vi "IVCurvePulsed.vi"(5 "XYGraph Refnum":refnum<vi>, 6 "Status":refnum<vi>, 7 "Source Code":string="-- The local functions are scoped at the project level, so that we can keep\n-- track of the reading buffers throughout the test.\nreset()\nsmua.reset()\nlocal systemNodes = {}\nlocal systemSmus = {}\nlocal systemSmuReadingBufferIndexes = {}\nlocal appendMode = 1\nlocal rangei = 1e-3\nlocal doCap =0\nlocal gOverrunDetected = false\n-- ==========================================================================\n-- This function tests for overruns in any of the system smus' trigger models.\n-- It returns an error to the application that will be displayed in a\n-- dialog box if an overrun occurs.\n-- ==========================================================================\nlocal _Overruncheck = function()\n    -- ==========================================================================\n    -- This function test the results of the value in the smu's trigger overrun\n    -- status register. -- It returns an error if an overrun occurs.\n    --\n    -- parameter   overrun     A bit pattern that contains the smu trigger overrun\n    --                         status register result\n    -- ==========================================================================\n    local TestOverrunBits = function(overrun, selNode, whichSmu)\n        local whichNode = [[localnode.]]\n        if (selNode.tsplink.node ~= localnode.tsplink.node) then\n            whichNode = [[node[]] .. selNode.tsplink.node .. [[].]]\n        end\n        whichNode = whichNode .. whichSmu .. [[ (]] .. selNode.model .. [[)]]\n        if (bit.test(overrun, 2)) then\n            gOverrunDetected = true\n            return (\"arm overrun on \" .. whichNode .. \"{eol}\")\n        elseif (bit.test(overrun, 3)) then\n            gOverrunDetected = true\n            return (\"source overrun on \" .. whichNode .. \"{eol}\")\n        elseif (bit.test(overrun, 4)) then\n            gOverrunDetected = true\n            return (\"measure overrun on \" .. whichNode .. \"{eol}\")\n        elseif (bit.test(overrun, 5)) then\n            gOverrunDetected = true\n            return (\"end pulse overrun on \" .. whichNode .. \"{eol}\")\n        else\n            return (\"\")\n        end\n    end\n\n    -- Report an overrun error only once.\n    if (gOverrunDetected == false) then\n        local allSmusInOverrun = [[]]\n\n        for i, selNode in ipairs(systemNodes) do\n            for j, selSmu in ipairs(systemSmus[i]) do\n                if (j == 1) then\n                    local overrun = selNode.status.operation.instrument.smua.trigger_overrun.event\n                    if (overrun > 0) then\n                        allSmusInOverrun = allSmusInOverrun .. TestOverrunBits(overrun, selNode, [[smua]])\n                    end\n                elseif (j == 2) then\n                    local overrun = selNode.status.operation.instrument.smub.trigger_overrun.event\n                    if (overrun > 0) then\n                        allSmusInOverrun = allSmusInOverrun .. TestOverrunBits(overrun, selNode, [[smub]])\n                    end\n                end\n            end\n        end\n\n        if (gOverrunDetected == true) then\n            print(\"[{error}]Script stopped due to:{eol}\" .. allSmusInOverrun)\n        end\n    end\nend\n\nlocal gComplianceDetected = false\n-- ==========================================================================\n-- Checks smus for voltage or current compliance.\n-- If a compliance event occurs, the message dialog box is presented to the\n-- user.\n-- ==========================================================================\nlocal _ComplianceCheck = function()\n    -- Report a compliance error only once.\n    if (gComplianceDetected == false) then\n        local allSmusInCompliance = [[]]\n\n        for i, selNode in ipairs(systemNodes) do\n            for j, selSmu in ipairs(systemSmus[i]) do\n                local compDetect = selNode.status.measurement.instrument.event\n                if (compDetect > 0) then\n                    -- Compose and show error message\n                    local whichNode = [[localnode.]]\n                    if (selNode.tsplink.node ~= localnode.tsplink.node) then\n                        whichNode = [[node[]] .. selNode.tsplink.node .. [[].]]\n                    end\n                    local whichSmu = [[]]\n                    if (compDetect == 2) then\n                        whichSmu = whichNode .. [[smua]]\n                    elseif (compDetect == 4) then\n                        whichSmu = whichNode .. [[smub]]\n                    elseif (compDetect == 6) then\n                        whichSmu = whichNode .. [[smua and ]] .. whichNode .. [[smub]]\n                    end\n                    whichSmu = whichSmu .. [[ (]] .. selNode.model .. [[){eol}]]\n                    allSmusInCompliance = allSmusInCompliance .. whichSmu\n\n                    -- Set gComplianceDetected so we don't report the error again.\n                    gComplianceDetected = true\n                end\n            end\n        end\n\n        if (gComplianceDetected == true) then\n            print(\"[{info}]Compliance detected on:{eol}\" .. allSmusInCompliance ..\n                      \"{eol}Click the Advanced button and check the Source Limit setting.\")\n        end\n    end\nend\n\nlocal gTestAborted = false\n-- ==========================================================================\n-- This function waits up to a specified period for the sweeps to complete.\n-- If the delay parameter is -1, then the timeout is infinite. It returns true\n-- if all sweeping actions are complete. Otherwise, the return value is false.\n-- Note: If gTestAborted is true, this function returns false immediately.\n--\n-- parameter  interval     Maximum time to wait (in seconds).\n-- ==========================================================================\nlocal _WaitForComplete = function(interval)\n    local pollInterval = 0.1\n\n    -- ==========================================================================\n    -- Checks the system smus for any that are still sweeping.\n    -- ==========================================================================\n    local IsSweepingComplete = function()\n        for i, selNode in ipairs(systemNodes) do\n            for j, selSmu in ipairs(systemSmus[i]) do\n                if (j == 1) then\n                    local statcond = selNode.status.operation.instrument.smua.condition\n                    if (bit.test(statcond, 4)) then\n                        return false\n                    end\n                elseif (j == 2) then\n                    local statcond = selNode.status.operation.instrument.smub.condition\n                    if (bit.test(statcond, 4)) then\n                        return false\n                    end\n                end\n            end\n        end\n\n        return true\n    end\n\n    local notimeout = false\n    if (interval < 0) then\n        notimeout = true\n        interval = 1\n    end\n\n    while (interval > 0) do\n        -- Check the abort flag\n        if (gTestAborted == true) then\n            return false\n        end\n\n        -- Check for errors\n        if (errorqueue.count > 0) then\n            return false\n        end\n\n        -- Check for overruns and compliance\n        _Overruncheck()\n        _ComplianceCheck()\n\n        if (IsSweepingComplete() == true) then\n            return true\n        end\n\n        delay(pollInterval)\n\n        if (notimeout == false) then\n            interval = interval - pollInterval\n        end\n    end\n\n    if (IsSweepingComplete() == true) then\n        return true\n    end\n\n    return false\nend\n----------------------------------------------------------------------------\n-- START OF INITIALIZE SEGMENT ... do not modify this section\n----------------------------------------------------------------------------\n-- ==========================================================================\n-- This function prepares the test for execution. \n-- It first verifies that current setup matches project's setup. \n-- Then, it initializes members used to keep track of reading buffer storage.\n-- ==========================================================================\nfunction _Initialize()\n    local maxNodes = 64 -- Maximum possible nodes in TSP link system.\n\n    local projectSetup = {{localnode, [[2636A]], [[2.2.1]]}} -- Instrument configuration for the project.\n    local currentSetup = {} -- Current instrument configuration.\n\n    local errorTag = \"[{error}]\"\n    local errorMessage = {[[Instrument in project configuration not found.]],\n                          [[Instrument configuration at does not match.]]}\n    local errorNo = 0\n\n    -- ==========================================================================\n    -- Configures the status model to detect voltage or current compliance.\n    -- ==========================================================================\n    local ConfigStatusModel = function()\n        for i, selNode in ipairs(systemNodes) do\n            selNode.status.reset()\n            for j, selSmu in ipairs(systemSmus[i]) do\n                -- The selSmu.source.compliance call will force an update\n                -- the condition register of the measurement.instrument.smuX to\n                -- update\n                local dum = selSmu.source.compliance\n                if (j == 1) then\n                    -- Clear the measurement.instrument.smua event register by reading its value\n                    dum = selNode.status.measurement.instrument.smua.event\n                    -- Now configure the status model to detect voltage or current compliance\n                    selNode.status.measurement.instrument.smua.enable = 3\n                    selNode.status.measurement.instrument.smua.ptr = 3\n                    selNode.status.measurement.instrument.enable = 6\n                    selNode.status.measurement.instrument.ptr = 6\n                elseif (j == 2) then\n                    -- Clear the measurement.instrument.smub event register by reading its value\n                    dum = selNode.status.measurement.instrument.smub.event\n                    -- Now configure the status model to detect voltage or current compliance\n                    selNode.status.measurement.instrument.smub.enable = 3\n                    selNode.status.measurement.instrument.smub.ptr = 3\n                end\n            end\n        end\n    end\n\n    -- ==========================================================================\n    -- Determines the current system configuration.\n    -- ==========================================================================\n    local GetSetup = function()\n        local masterNode = tsplink.node\n\n        systemSmus = {}\n        systemNodes = {}\n        systemNodes[1] = node[masterNode]\n\n        currentSetup[1] = {}\n        currentSetup[1][1] = node[masterNode]\n        currentSetup[1][2] = node[masterNode].model\n        currentSetup[1][3] = node[masterNode].revision\n\n        systemSmus[1] = {}\n        systemSmus[1][1] = node[masterNode].smua\n\n        if (node[masterNode].smub ~= nil) then\n            systemSmus[1][2] = node[masterNode].smub\n        end\n\n        local j = 2\n        for i = 1, maxNodes do\n            if ((tsplink.node ~= i) and (node[i] ~= nil)) then\n                systemNodes[j] = node[i]\n                currentSetup[j] = {}\n                currentSetup[j][1] = node[i]\n                currentSetup[j][2] = node[i].model\n                currentSetup[j][3] = node[i].revision\n\n                systemSmus[j] = {}\n                systemSmus[j][1] = node[i].smua\n\n                if (node[i].smub ~= nil) then\n                    systemSmus[j][2] = node[i].smub\n                end\n                j = j + 1\n            end\n        end\n    end\n\n    GetSetup()\n\n    -- Check the project setup versus the configuration setup.\n    -- If there is a difference, report an error.\n    local numpInstruments = table.getn(projectSetup)\n    local numcInstruments = table.getn(currentSetup)\n\n    for i = 1, numpInstruments do\n        local pfields = table.getn(projectSetup[i])\n\n        errorNo = 1\n        for j = 1, numcInstruments do\n            -- Compare nodes.\n            if (projectSetup[i][1] == currentSetup[j][1]) then\n                errorNo = 0\n\n                for k = 2, pfields do\n                    if (projectSetup[i][k] ~= currentSetup[j][k]) then\n                        errorNo = 2\n                    end\n                end\n                break\n            end\n        end\n\n        if (errorNo > 0) then\n            break\n        end\n    end\n\n    if (errorNo > 0) then\n        error(errorMessage[errorNo])\n        print(errorTag .. errorMessage[errorNo])\n    end\n\n    -- ==========================================================================\n    -- Initializes all system readings buffers by clearing and setting them to\n    -- append mode. An array, sysSmuReadingBufferIndexes, is used to keep track of the\n    -- data stored to each of the reading buffers.\n    -- ==========================================================================\n    local InitalizeReadingBuffers = function()\n        systemSmuReadingBufferIndexes = {}\n        for i, selNode in ipairs(systemSmus) do\n            systemSmuReadingBufferIndexes[i] = {}\n\n            for j, selSmu in ipairs(selNode) do\n                -- Create an array for the smu.\n                systemSmuReadingBufferIndexes[i][j] = {}\n\n                local snvBuffers = {selSmu.nvbuffer1, selSmu.nvbuffer2}\n                for k, selBuffer in ipairs(snvBuffers) do\n                    -- Create an array for nvbuffers 1 and 2.\n                    systemSmuReadingBufferIndexes[i][j][k] = {}\n\n                    local sysSmuReadingBufferIndexes = systemSmuReadingBufferIndexes[i][j][k]\n                    sysSmuReadingBufferIndexes[\"start\"] = 0\n                    sysSmuReadingBufferIndexes[\"stop\"] = 0\n\n                    selBuffer.clear()\n                    selBuffer.appendmode = 1\n                    selBuffer.collecttimestamps = 1\n                    selBuffer.collectsourcevalues = 1\n                    selBuffer.timestampresolution = 1e-6\n                    if (selBuffer.fillmode ~= nil) then\n                        selBuffer.fillmode = selSmu.FILL_ONCE\n                    end\n                end\n\n            end\n        end\n    end\n\n    InitalizeReadingBuffers()\n    ConfigStatusModel()\nend\n----------------------------------------------------------------------------\n-- END OF INITIALIZE SEGMENT ... do not modify code after this point\n----------------------------------------------------------------------------\n\n----------------------------------------------------------------------------\n-- START OF SWEEP SEGMENT ... do not modify this section\n----------------------------------------------------------------------------\n-- ==========================================================================\n-- Configures a sweeping test.\n-- (This represents a Sweep segment of the script.  Click on the Sweep tab to customize it.)\n-- ==========================================================================\nfunction _Sweep()\n    local highSpeedSampling = false\n    local errorTag = \"[{error}]\"\n    local biasIndex = 1\n    local stepIndex = 2\n    local sweepIndex = 3\n    local numLevels = 3\n    local nvBuffersUsed = {1, 1, 1}\n    -- local alias for SMUs\n    local sweep1 = localnode.smua -- is a 2636A\n    -- \"NoStepFixed\" configuration (autorange enabled = false,  #step channels = 0):\n    -- This function configures any number of sweeping smus with no stepping smus.\n    -- It supports sweeps with autorange off and pulse mode.\n    local testSmus = {{{}}, -- Bias\n    {{}}, -- Step\n    {{localnode.smua}} -- Sweep\n    }\n\n    local testNodes = {{}, -- Bias\n    {}, -- Step\n    {localnode} -- Sweep\n    }\n\n    local sweepPulseModes = {{false}}\n\n    local timePoint = 0.1\n    local pulseWidth = 99.0000009537E-3\n    local measurePointTime = 16.7266666667E-3\n\n    local numberOfSteps = 1\n    local numberOfSweeps = #NumPoints\n\n    local nplc = 1\n    local lineFrequency = 60\n\n    local numNodes = table.getn(testNodes[sweepIndex])\n    local numMasterSmus = table.getn(testSmus[sweepIndex][1])\n    local masterNode = testNodes[sweepIndex][1]\n    local masterSweepSmu = testSmus[sweepIndex][1][1]\n\n    local t1Timer = masterNode.trigger.timer[1] -- t1Timer is for sweep time per point\n    local t2Timer = masterNode.trigger.timer[2] -- t2Timer is for sweep pulse width\n    local t3Timer = masterNode.trigger.timer[3] -- t3Timer is for a 1ms initial delay\n\n    local masterTspLine1 = masterNode.tsplink.trigger[1] -- for source stimulus\n    local masterTspLine2 = masterNode.tsplink.trigger[2] -- for endpulse stimulus\n\n    -- ==========================================================================\n    -- This function checks for errors or conflicts in the test settings (timing, ranges, etc.)\n    -- ==========================================================================\n    local CheckSettings = function()\n        local measureDelay = timePoint - measurePointTime\n\n        local errorMsg = nil\n\n        -- Valid timing paramaters\n        -- None of these errors should appear to the user.\n        if (masterSweepSmu == nil) then\n            errorMsg = [[Must have at least one sweeping smu.]]\n        elseif (timePoint <= 0) then\n            errorMsg = [[timePoint <= 0]]\n        elseif (pulseWidth <= 0) then\n            errorMsg = [[pulseWidth <= 0]]\n        elseif (pulseWidth > timePoint) then\n            errorMsg = [[pulseWidth > timePoint]]\n        elseif (measureDelay < 0) then\n            errorMsg = [[timePoint too small, <= measurePointTime]]\n        end\n\n        if (errorMsg ~= nil) then\n            print(errorTag .. errorMsg)\n            error(errorMsg)\n        end\n    end\n\n    -- ==========================================================================\n    -- This function configures the trigger line interaction between the smus.\n    -- ==========================================================================\n    local ConfigureTriggerLines = function()\n        -- ==========================================================================\n        -- This function configures the timers that are used in the test.\n        -- ==========================================================================\n        local ConfigureSweepTimers = function()\n            -- t3Timer provides a 1ms initial delay following the masterSweepSmu's armed event ID.\n            -- This is to ensure that masterSweepSmu is fully ready for the first source stimulus.\n            t3Timer.stimulus = masterSweepSmu.trigger.ARMED_EVENT_ID\n            t3Timer.passthrough = false\n            t3Timer.delay = 1.0e-3\n            t3Timer.count = 1\n\n            if (numberOfSweeps > 1) then\n                t1Timer.stimulus = t3Timer.EVENT_ID\n                t1Timer.passthrough = true\n                t1Timer.delay = timePoint\n                t1Timer.count = numberOfSweeps - 1\n\n                t2Timer.stimulus = t1Timer.EVENT_ID\n            else\n                -- Cannot use t1Timer when numberOfSweeps <= 1\n                t2Timer.stimulus = t3Timer.EVENT_ID\n            end\n\n            t2Timer.passthrough = false\n            t2Timer.delay = pulseWidth\n            t2Timer.count = 1\n        end\n\n        -- ==========================================================================\n        -- This function configures the sweeping smus.\n        -- ==========================================================================\n        local ConfigureSweep = function()\n\n            -- ==========================================================================\n            -- This function configures all sweeping smus on the master node.\n            -- ==========================================================================\n            local ConfigureMasterNodeSweepSmus = function()\n                for i = 1, numMasterSmus do\n                    local pulseMode = sweepPulseModes[1][i]\n                    local selSmu = testSmus[sweepIndex][1][i]\n                    local sourceStimulus = masterTspLine1.EVENT_ID\n\n                    if (i == 1) then\n                        -- masterSweepSmu will be triggered by StartSweep()\n                        -- Use a dummy event ID as a place holder for the arm stimulus\n                        selSmu.trigger.arm.stimulus = masterNode.trigger.EVENT_ID\n                    else\n                        selSmu.trigger.arm.stimulus = 0\n                    end\n\n                    selSmu.trigger.source.stimulus = sourceStimulus\n                    selSmu.trigger.source.action = selSmu.ENABLE\n\n                    if ((pulseMode == true) and (pulseWidth < timePoint)) then\n                        selSmu.trigger.endpulse.stimulus = masterTspLine2.EVENT_ID\n                        selSmu.trigger.endpulse.action = selSmu.SOURCE_IDLE\n                    else\n                        selSmu.trigger.endpulse.stimulus = selSmu.trigger.MEASURE_COMPLETE_EVENT_ID\n                        selSmu.trigger.endpulse.action = selSmu.SOURCE_HOLD\n                    end\n\n                    if (highSpeedSampling == true) then\n                        selSmu.trigger.measure.stimulus = sourceStimulus\n                        selSmu.trigger.measure.action = selSmu.ASYNC\n\n                        -- Cannot collect source values when in asynchronous mode\n                        selSmu.nvbuffer1.collectsourcevalues = 0\n                        selSmu.nvbuffer2.collectsourcevalues = 0\n                    else\n                        selSmu.trigger.measure.stimulus = 0\n                        selSmu.trigger.measure.action = selSmu.ENABLE\n                    end\n\n                    selSmu.trigger.arm.count = numberOfSteps\n                    selSmu.trigger.count = numberOfSweeps\n                end\n            end\n\n            -- ==========================================================================\n            -- This function configures a sweeping smu on a remote node\n            --\n            -- parameter pulseMode      true for Pulse mode,  false otherwise.\n            -- parameter selNode        Node to which the smu belongs.\n            -- parameter selSmu         Smu to configure.\n            -- ==========================================================================\n            local ConfigureRemoteSweepSmu = function(pulseMode, selNode, selSmu)\n                local tspl1 = selNode.tsplink.trigger[1]\n                local tspl2 = selNode.tsplink.trigger[2]\n                local sourceStimulus = tspl1.EVENT_ID\n\n                selSmu.trigger.arm.stimulus = 0\n                selSmu.trigger.source.stimulus = sourceStimulus\n                selSmu.trigger.source.action = selSmu.ENABLE\n\n                if ((pulseMode == true) and (pulseWidth < timePoint)) then\n                    selSmu.trigger.endpulse.stimulus = tspl2.EVENT_ID\n                    selSmu.trigger.endpulse.action = selSmu.SOURCE_IDLE\n                else\n                    selSmu.trigger.endpulse.stimulus = selSmu.trigger.MEASURE_COMPLETE_EVENT_ID\n                    selSmu.trigger.endpulse.action = selSmu.SOURCE_HOLD\n                end\n\n                if (highSpeedSampling == true) then\n                    selSmu.trigger.measure.stimulus = sourceStimulus\n                    selSmu.trigger.measure.action = selSmu.ASYNC\n\n                    -- Cannot collect source values when in asynchronous mode\n                    selSmu.nvbuffer1.collectsourcevalues = 0\n                    selSmu.nvbuffer2.collectsourcevalues = 0\n                else\n                    selSmu.trigger.measure.stimulus = 0\n                    selSmu.trigger.measure.action = selSmu.ENABLE\n                end\n\n                selSmu.trigger.arm.count = numberOfSteps\n                selSmu.trigger.count = numberOfSweeps\n            end\n\n            -- ===========================\n            -- START of ConfigureSweep()\n            -- ===========================\n            -- Prepare a tsplink trigger line for source stimulus on the master node\n            masterTspLine1.mode = tsplink.TRIG_FALLING\n            masterTspLine1.pulsewidth = 1e-6\n            if (numberOfSweeps > 1) then\n                masterTspLine1.stimulus = t1Timer.EVENT_ID\n            else\n                masterTspLine1.stimulus = t3Timer.EVENT_ID\n            end\n\n            -- Prepare a tsplink trigger line for endpulse stimulus on the master node\n            masterTspLine2.mode = tsplink.TRIG_FALLING\n            masterTspLine2.pulsewidth = 1e-6\n            masterTspLine2.stimulus = t2Timer.EVENT_ID\n\n            -- Configure all sweep smus on the master node.\n            -- The master node contains the smu that kicks off the sweeps.\n            ConfigureMasterNodeSweepSmus()\n\n            -- Configure the sweeping smus on remote nodes\n            if (numNodes > 1) then\n                for i = 2, numNodes do\n                    -- For each remote node, configure the tsplink trigger lines\n                    local selNode = testNodes[sweepIndex][i]\n\n                    local tspl1 = selNode.tsplink.trigger[1]\n                    tspl1.mode = tsplink.TRIG_FALLING\n                    tspl1.pulsewidth = 1e-6\n                    tspl1.stimulus = 0\n\n                    local tspl2 = selNode.tsplink.trigger[2]\n                    tspl2.mode = tsplink.TRIG_FALLING\n                    tspl2.pulsewidth = 1e-6\n                    tspl2.stimulus = 0\n\n                    local sweepSmus = testSmus[sweepIndex]\n                    local numSmus = table.getn(sweepSmus[i])\n\n                    for j = 1, numSmus do\n                        -- For each sweeping smu on each remote node, configure the remote sweeping smu\n                        local extSmu = sweepSmus[i][j]\n                        local pulseMode = sweepPulseModes[i][j]\n\n                        ConfigureRemoteSweepSmu(pulseMode, selNode, extSmu)\n                    end\n                end\n            end\n        end\n\n        -- Configure timers and sweep trigger lines.\n        ConfigureSweepTimers()\n        ConfigureSweep()\n    end\n\n    -- ==========================================================================\n    -- This function kicks off the sweep.\n    -- ==========================================================================\n    local StartSweep = function()\n        masterSweepSmu.trigger.arm.set()\n    end\n    -- ==========================================================================\n    -- Resets all components that may be used in the test.\n    -- ==========================================================================\n    local Reset = function()\n        for i, selTest in ipairs(testSmus) do\n            for j, selNode in ipairs(testNodes[i]) do\n                if (selNode ~= nil) then\n                    -- Reset blenders\n                    local k = 1\n                    while (selNode.tsplink.trigger[k] ~= nil) do\n                        selNode.tsplink.trigger[k].reset()\n                        k = k + 1\n                    end\n\n                    k = 1\n                    while (selNode.trigger.blender[k] ~= nil) do\n                        selNode.trigger.blender[k].reset()\n                        k = k + 1\n                    end\n\n                    -- Reset Timers\n                    k = 1\n                    while (selNode.trigger.timer[k] ~= nil) do\n                        selNode.trigger.timer[k].reset()\n                        k = k + 1\n                    end\n                end\n            end\n\n            -- Reset Smus\n            for j, selNode in ipairs(selTest) do\n                for k, selSmu in ipairs(selNode) do\n                    if (selSmu ~= nil) then\n                        -- Resets all smus in the test.\n                        selSmu.reset()\n                    end\n                end\n            end\n        end\n    end\n\n    -- ==========================================================================\n    -- Turns all smus in the test on.\n    -- ==========================================================================\n    local TurnSmusOn = function()\n        for i, selTest in ipairs(testSmus) do\n            for j, selNode in ipairs(selTest) do\n                for k, selSmu in ipairs(selNode) do\n                    if (selSmu ~= nil) then\n                        if (selSmu.source.output ~= 1) then\n                            selSmu.source.output = 1\n                        end\n                    end\n                end\n            end\n        end\n    end\n\n    -- ==========================================================================\n    -- This function initiates the steping and sweeping smus.\n    -- ==========================================================================\n    local InitiateSmus = function()\n        for i = 2, numLevels do\n            for j, selNode in ipairs(testSmus[i]) do\n                for k, selSmu in ipairs(selNode) do\n                    if (selSmu ~= nil) then\n                        selSmu.trigger.initiate()\n                    end\n                end\n            end\n        end\n    end\n\n    -- ==========================================================================\n    -- This function determines the number of points that will be in the buffer at the end of the test.\n    -- ==========================================================================\n    local StoreReadingBufferIndexes = function()\n        -- ==========================================================================\n        -- Determines reading buffer starting and stopping indexes.\n        -- parameter    testLevel    Index referring to bias, step, or sweep.\n        -- parameter    i            Node index.\n        -- parameter    selSmuIndex  Selected smu index.\n        -- ==========================================================================\n        local SetupLastPoints = function(testLevel, i, selSmuIndex)\n            local stoppingPoint1 = 0\n            local stoppingPoint2 = 0\n            local incVal = 0\n            local selSmuRbIndex1 = systemSmuReadingBufferIndexes[i][selSmuIndex][1]\n            local selSmuRbIndex2 = systemSmuReadingBufferIndexes[i][selSmuIndex][2]\n\n            selSmuRbIndex1[\"start\"] = 1\n            selSmuRbIndex2[\"start\"] = 1\n\n            -- appendMode is a local variable common to the script.\n            if (appendMode == 1) then\n                stoppingPoint1 = selSmuRbIndex1[\"stop\"]\n                stoppingPoint2 = selSmuRbIndex2[\"stop\"]\n            end\n            -- Bias setup\n            if (testLevel == biasIndex) then\n                incVal = 1\n                -- Step setup\n            elseif (testLevel == stepIndex) then\n                incVal = (1 * 1)\n                -- Sweep setup\n            elseif (testLevel == sweepIndex) then\n                if (highSpeedSampling == true) then\n                    incVal = (1 * 200 * 60)\n                else\n                    incVal = (1 * 200 * 1)\n                end\n            end\n\n            selSmuRbIndex1[\"stop\"] = stoppingPoint1 + incVal\n            if (nvBuffersUsed[testLevel] == 2) then\n                selSmuRbIndex2[\"stop\"] = stoppingPoint2 + incVal\n            end\n        end\n\n        for i, selTest in ipairs(testSmus) do\n            for j, selNode in ipairs(selTest) do\n                for k, selSmu in ipairs(selNode) do\n                    for l, selSysNode in ipairs(systemSmus) do\n                        if (selSysNode[1] == selSmu) then\n                            SetupLastPoints(i, l, 1)\n                        end\n\n                        if (selSysNode[2] ~= nil) then\n                            if (selSysNode[2] == selSmu) then\n                                SetupLastPoints(i, l, 2)\n                            end\n                        end\n                    end\n                end\n            end\n        end\n    end\n    ---==========================================================================\n    -- The following makes sure we capture a measurement from the bias channels\n    -- ==========================================================================\n    local MeasureBiasChannels = function()\n    end\n    -- ==========================================================================\n    -- This function Configures the smu options such as nplc, function, range, etc.\n    -- ==========================================================================\n    local ConfigureSmus = function(rangei)\n        -- set up Sweep (inner sweep) for sweep1\n        sweep1.sense = sweep1.SENSE_LOCAL\n        sweep1.source.delay = 0\n        sweep1.measure.nplc = nplc\n        sweep1.measure.autozero = sweep1.AUTOZERO_OFF\n        sweep1.measure.count = 1\n        sweep1.measure.filter.enable = sweep1.FILTER_OFF\n        sweep1.measure.filter.type = sweep1.FILTER_MOVING_AVG\n        sweep1.measure.filter.count = 1\n        sweep1.measure.delay = 0\n        sweep1.measure.delayfactor = 1\n        sweep1.measure.analogfilter = 0\n        sweep1.source.func = sweep1.OUTPUT_DCVOLTS\n        if sweep1.source.highc == sweep1.ENABLE then\n            sweep1.source.highc = sweep1.DISABLE\n        end\n        sweep1.source.limiti = 10E-3\n        sweep1.trigger.source.limiti = sweep1.LIMIT_AUTO\n        sweep1.source.autorangev = 0\n        sweep1.source.rangev = 2\n        sweep1.trigger.source.listv({#VoltList})\n        sweep1.measure.autorangei = 0\n        sweep1.measure.rangei = rangei -- 100E-12\n        sweep1.measure.autorangev = sweep1.source.autorangev\n        if (sweep1.measure.autorangev == 0) then\n            sweep1.measure.rangev = sweep1.source.rangev\n        end\n        sweep1.trigger.measure.iv(sweep1.nvbuffer1, sweep1.nvbuffer2)\n        nvBuffersUsed[sweepIndex] = 2\n    end\n    -- Test starts here.\n\n    -- Make sure previous test is done.\n\n    _WaitForComplete(-1)\n\n    CheckSettings()\n    Reset()\n\n    smua.source.limiti = 1e-3\n    smua.source.levelv = .001\n    smua.source.output = 1\n    delay(.1)\n    local reading = smua.measure.i() * 2000\n\n    if (reading < rangei) then\n        rangei = rangei / 100\n        smua.source.output = 1\n        smua.source.limiti = 1e-3\n        smua.measure.rangei = rangei\n        smua.source.levelv = .001\n        delay(.1)\n        reading = smua.measure.i() * 2000\n        if (reading < rangei) then\n            rangei = rangei / 100\n            smua.source.output = 1\n            smua.source.limiti = 1e-3\n            smua.measure.rangei = rangei\n            smua.source.levelv = .001\n            delay(.1)\n            reading = smua.measure.i() * 2000\n            if (reading < rangei) then\n                rangei = rangei / 1000\n                doCap =1\n                smua.source.levelv = 0\n            end\n        end\n    end\n\n    ConfigureSmus(rangei)\n    ConfigureTriggerLines()\n\n    StoreReadingBufferIndexes()\n    TurnSmusOn()\n    MeasureBiasChannels()\n    smua.source.levelv = 0\n\n    InitiateSmus()\n    delay(1)\n    StartSweep()\nend\n----------------------------------------------------------------------------\n-- END OF SWEEP SEGMENT ... do not modify code after this point\n----------------------------------------------------------------------------\n\n----------------------------------------------------------------------------\n-- START OF DATAREPORT SEGMENT ... do not modify this section\n----------------------------------------------------------------------------\n-- ==========================================================================\n-- This script returns a series of reading buffers. \n-- (This represents a DataReport segment of the script.  Click on the Data tab to customize it.)\n-- ==========================================================================\nfunction _Data()\n    local buffers = {localnode.smua.nvbuffer1, localnode.smua.nvbuffer2} -- Array of reading buffers to return\n    local bufferNames = {[[localnode.smua.nvbuffer1]], [[localnode.smua.nvbuffer2]]} -- Array of reading buffer names\n    local bufferSmuNames = {[[Sweep_SMU]], [[Sweep_SMU]]} -- Array of SMU names for each reading buffer\n    local expectedCount = {} -- Array containing the expected number of return values.\n    local waitInterval = 1 -- Interval between message transfers\n    local maxToReturn = 100 -- Maximum reading buffer points between message transfers.\n\n    -- The following are special tokens used internally by the data report function\n    local DATA_REPORT = \"(({{Data}}))\"\n    local SWEEPSTART = \"{SWEEP-START}\"\n    local START = \"{START}\"\n    local NAME = \"{NAME}\"\n    local EXPECTED_COUNT = \"{EXPECTED-COUNT}\"\n    local PTS_IN_BUFF = \"{PTS-IN-BUFF}\"\n    local PTS_RETURNED = \"{PTS-RETURNED}\"\n    local BASE_TIME_STAMP = \"{BASE-TIME-STAMP}\"\n    local READINGS = \"{READINGS}\"\n    local TIMESTAMPS = \"{TIMESTAMPS}\"\n    local SRCVALS = \"{SRCVALS}\"\n    local END = \"{END}\"\n    local COMPLETE = \"{COMPLETE}\"\n\n    local errorTag = \"[{error}]\"\n    local dataIndexes = {} -- Data transfer index for each reading buffer\n    local done = true -- True when data transfer from all of reading buffers is completed\n    local dataComplete = true -- True when all of reading buffers have reached their expected counts\n\n    -- ==========================================================================\n    -- This function determines the ending points that will be in the buffer\n    -- at the time data collection takes place.\n    -- ==========================================================================\n    local GetStopPoints = function()\n        for i, selBuffer in ipairs(buffers) do\n            for j, selSysNode in ipairs(systemSmus) do\n                for k, selSmu in ipairs(selSysNode) do\n                    if (selSmu.nvbuffer1 == selBuffer) then\n                        expectedCount[i] = systemSmuReadingBufferIndexes[j][k][1][\"stop\"]\n                    elseif (selSmu.nvbuffer2 == selBuffer) then\n                        expectedCount[i] = systemSmuReadingBufferIndexes[j][k][2][\"stop\"]\n                    end\n                end\n            end\n        end\n    end\n\n    -- ==========================================================================\n    -- Checks if the SMU for selBuffer is sweeping.\n    -- ==========================================================================\n    local IsSweeping = function(selBuffer)\n        for i, selNode in ipairs(systemNodes) do\n            for j, selSmu in ipairs(systemSmus[i]) do\n                if (j == 1) then\n                    if ((selSmu.nvbuffer1 == selBuffer) or (selSmu.nvbuffer2 == selBuffer)) then\n                        local statcond = selNode.status.operation.instrument.smua.condition\n                        return (bit.test(statcond, 4)) -- Check Bit B3, Sweeping (SWE)\n                    end\n                elseif (j == 2) then\n                    if ((selSmu.nvbuffer1 == selBuffer) or (selSmu.nvbuffer2 == selBuffer)) then\n                        local statcond = selNode.status.operation.instrument.smub.condition\n                        return (bit.test(statcond, 4)) -- Check Bit B3, Sweeping (SWE)\n                    end\n                end\n            end\n        end\n        return false\n    end\n\n    -- ==========================================================================\n    -- Clears the reading buffers and resets the array that contains the\n    -- reading buffer storage start/ stop points.\n    -- ==========================================================================\n    local ClearReturnedBuffers = function()\n        for i, selBuffer in ipairs(buffers) do\n            selBuffer.clear()\n\n            local smuBufferIndex = nil\n            for j, selSysNode in ipairs(systemSmus) do\n                for k, selSmu in ipairs(selSysNode) do\n                    if (selSmu.nvbuffer1 == selBuffer) then\n                        smuBufferIndex = systemSmuReadingBufferIndexes[j][k][1]\n                    elseif (selSmu.nvbuffer2 == selBuffer) then\n                        smuBufferIndex = systemSmuReadingBufferIndexes[j][k][2]\n                    end\n                end\n            end\n            if (smuBufferIndex ~= nil) then\n                smuBufferIndex[\"start\"] = 0\n                smuBufferIndex[\"stop\"] = 0\n            end\n        end\n    end\n\n    GetStopPoints()\n\n    -- Initialize dataIndex. This array is used to keep track of the points returned to\n    -- the application.\n\n    for i, v in ipairs(buffers) do\n        dataIndexes[i] = 1\n    end\n\n    -- The following print statements turns on data report feature within the application.\n\n    repeat\n        done = true\n        dataComplete = true\n        for i, selBuffer in ipairs(buffers) do\n            -- Check for smu trigger model overruns.\n            _Overruncheck()\n\n            -- Check for smu compliance.\n            _ComplianceCheck()\n\n            -- Caution: Check for stillSweeping BEFORE getting numPointsStored\n            local stillSweeping = IsSweeping(selBuffer)\n            local numPointsStored = selBuffer.n\n\n            -- Check for sweep completion before data is complete (i.e. something bad happened)\n            if ((numPointsStored < expectedCount[i]) and (stillSweeping == false)) then\n                gTestAborted = true\n            end\n\n            dataComplete = dataComplete and (numPointsStored >= expectedCount[i])\n            done = done and (dataIndexes[i] > expectedCount[i])\n\n            if (dataIndexes[i] <= numPointsStored) then\n                local points = numPointsStored - dataIndexes[i] + 1\n\n                if (points > maxToReturn) then\n                    points = maxToReturn\n                end\n\n                local retString = string.format(\"%d,%d,\", i, points)\n\n                local start = dataIndexes[i]\n                local stop = start + points - 1\n\n                local readings = \"\"\n\n                for j = start, stop do\n                    if (j == start) then\n                        readings = readings .. string.format(\"%e,\", selBuffer.readings[j])\n                    else\n                        readings = readings .. string.format(\"%e,\", selBuffer.readings[j])\n                    end\n                end\n\n                local timestamps = \"\"\n                if (selBuffer.collecttimestamps == 1) then\n                    for j = start, stop do\n                        if (j == start) then\n                            timestamps = timestamps .. string.format(\"%e,\", selBuffer.timestamps[j])\n                        else\n                            timestamps = timestamps .. string.format(\"%e,\", selBuffer.timestamps[j])\n                        end\n                    end\n                end\n\n                local srcValues = \"\"\n                if (selBuffer.collectsourcevalues == 1) then\n                    for j = start, stop do\n                        if (j == start) then\n                            srcValues = srcValues .. string.format(\"%e,\", selBuffer.sourcevalues[j])\n                        else\n                            srcValues = srcValues .. string.format(\"%e,\", selBuffer.sourcevalues[j])\n                        end\n                    end\n                end\n\n                dataIndexes[i] = stop + 1\n\n                print(string.format(\"%d,%d,\", i + 1, points) .. readings)\n                print(string.format(\"%d,%d,\", 0, points) .. timestamps)\n                print(string.format(\"%d,%d,\", 1, points) .. srcValues)\n\n            end\n        end\n\n        if (dataComplete == false) then\n            if (gTestAborted == true) then\n                done = true -- Stop waiting for data completion because it will never happen\n            else\n                delay(waitInterval)\n            end\n        end\n    until (done == true)\n\n    print(COMPLETE .. \"\\n\")\n\n    -- The application may not have selected all the buffers being used in the test, so\n    -- we need to make sure the overlapped operations are complete before clearing the buffers.\n    local sweepCompleted = _WaitForComplete(-1)\n\n    if (sweepCompleted == true) then\n        ClearReturnedBuffers()\n    end\nend\n----------------------------------------------------------------------------\n-- END OF DATAREPORT SEGMENT ... do not modify code after this point\n----------------------------------------------------------------------------\n\n----------------------------------------------------------------------------\n-- START OF FINALIZE SEGMENT ... do not modify this section\n----------------------------------------------------------------------------\n-- ==========================================================================\n-- The function completes the script and places the instrument in a known state.\n-- ==========================================================================\nfunction _Finalize()\n    -- Wait for test completion\n    local sweepCompleted = _WaitForComplete(-1)\n\n    -- Check for abnornal completion\n    if (sweepCompleted == false) then\n        -- Abort all overlapped operations on all smus\n        for i, selNode in ipairs(systemNodes) do\n            for j, selSmu in ipairs(systemSmus[i]) do\n                selSmu.abort()\n            end\n        end\n\n        -- Check for errors\n        if (errorqueue.count > 0) then\n            print(\"[{error}]Script stopped due to error(s).\")\n        else\n            print(\"[{error}]Script stopped before completion.\")\n        end\n    end\n\n    -- Set output level to 0V and 0A for all SMUs\n    for i, selNode in ipairs(systemNodes) do\n        for j, selSmu in ipairs(systemSmus[i]) do\n            selSmu.source.leveli = 0\n            selSmu.source.levelv = 0\n        end\n    end\n\n    -- Turn output off for all SMUs\n    for i, selNode in ipairs(systemNodes) do\n        for j, selSmu in ipairs(systemSmus[i]) do\n            selSmu.source.output = 0\n        end\n    end\n\n    -- Reset the system,  placing it into a known safe state.\n    reset()\nend\n----------------------------------------------------------------------------\n-- END OF FINALIZE SEGMENT ... do not modify code after this point\n----------------------------------------------------------------------------\n\n_Initialize()\n_Sweep()\n_Data()\n_Finalize()\n\n\n\n\nfunction AC_Waveform_Sweep(Vrms,VLin, numCycles, frequency, limitI,skips)\n\treset()\n\tlocal COMPLETE = \"{COMPLETE}\"\n\t-- Generate the source values\n\tlocal Vpp\t\t\t\t= Vrms * math.sqrt(2)\n\tlocal sourceValues\t\t= {} \n\tlocal pointsPerCycle\t= 7200 / frequency\n\tlocal numDataPoints\t\t= pointsPerCycle * numCycles\n\n\tlocal res = {}\n    local cap = {}\n    for i = 1, numDataPoints do\n        res[i] = math.sin(i * 2 * math.pi / pointsPerCycle)\n        cap[i] = math.cos(i * 2 * math.pi / pointsPerCycle)\n        sourceValues[i] = (Vpp * res[i]) + Vpp + VLin\n    end\n\n\t-- Configure the SMU ranges\n\tsmua.reset()\n\tsmua.source.settling\t\t= smua.SETTLE_FAST_POLARITY\n\tsmua.source.autorangev\t\t= smua.AUTORANGE_OFF\n\tsmua.source.autorangei\t\t= smua.AUTORANGE_OFF\n\tsmua.source.rangev\t\t\t= 2 * Vpp + VLin\n\tsmua.source.delay\t\t\t= 0\n\tsmua.source.limiti\t\t\t= 1e-3\n\n\tsmua.measure.autorangev\t\t= smua.AUTORANGE_OFF\n\tsmua.measure.autorangei\t\t= smua.AUTORANGE_OFF\n\tsmua.measure.autozero\t\t= smua.AUTOZERO_OFF\n\tsmua.measure.delay\t\t\t= 0\n\tsmua.measure.delayfactor    = 1\n\tsmua.measure.analogfilter   = 0\n\n\t-- Voltage will be measured on the same range as the source range\n\tsmua.measure.rangei\t\t\t= limitI\n\tsmua.measure.nplc\t\t\t= 0.001\n\n\t-- Prepare the Reading Buffers\n\tsmua.nvbuffer1.clear()\n\tsmua.nvbuffer1.collecttimestamps\t= 1\n\tsmua.nvbuffer2.clear()\n\tsmua.nvbuffer2.collecttimestamps\t= 1\n\n\t-- Configure the trigger model\n\t--============================\n\t\n\t-- Timer 1 controls the time between source points\n\ttrigger.timer[1].delay = (1 / 7200)\n\ttrigger.timer[1].passthrough = true\n\ttrigger.timer[1].stimulus = smua.trigger.ARMED_EVENT_ID\n\ttrigger.timer[1].count = numDataPoints - 1\n\n\t-- Configure the SMU trigger model\n\tsmua.trigger.source.listv(sourceValues)\n\tsmua.trigger.source.limiti\t\t= limitI\n\tsmua.trigger.measure.action\t\t= smua.ENABLE\n\tsmua.trigger.measure.iv(smua.nvbuffer1, smua.nvbuffer2)\n\tsmua.trigger.endpulse.action\t= smua.SOURCE_HOLD\n\tsmua.trigger.endsweep.action\t= smua.SOURCE_IDLE\n\tsmua.trigger.count\t\t\t\t= numDataPoints\n\tsmua.trigger.arm.stimulus\t\t= 0\n\tsmua.trigger.source.stimulus\t= trigger.timer[1].EVENT_ID\n\tsmua.trigger.measure.stimulus\t= 0\n\tsmua.trigger.endpulse.stimulus\t= 0\n\tsmua.trigger.source.action\t\t= smua.ENABLE\n\t-- Ready to begin the test\n\n\tsmua.source.output\t\t\t\t\t= smua.OUTPUT_ON\n\t-- Start the trigger model execution\n\tsmua.trigger.initiate()\n\t-- Wait until the sweep has completed\n\twaitcomplete()\n\tsmua.source.output\t\t\t\t\t= smua.OUTPUT_OFF\n\n\t-- Print the data back to the Console in tabular format\n    singleWave = {}\n\tvisits ={}\n\tsize1=0\n\tphaseC = 0\n    phaseS = 0\n    mid = 0\n    cc=0\n    for x=pointsPerCycle, smua.nvbuffer2.n do\n      \tlocal i = math.floor( x - math.floor(x/(pointsPerCycle))*(pointsPerCycle))\n\t\tv=\tsmua.nvbuffer1[x]\n\t\tif (math.abs(v)<1e-3) then\n            if (singleWave[i]==nil) then \n                singleWave[i]=v\n                visits[i]=1\n                if (size1<i) then size1=i end\n            else \n                singleWave[i]=singleWave[i]+v\n                visits[i]=visits[i]+ 1\n            end\t\n        end\n\t\tphaseC = phaseC + cap[x] * v\n        phaseS = phaseS + res[x] * v\n        mid = mid + v\n        cc=cc+1\n--\t    print(smua.nvbuffer1.timestamps[x], smua.nvbuffer2[x], smua.nvbuffer1[x])\n    end\n\n    mid = mid / cc\n    phaseC = 2 * phaseC / cc\n    phaseS = 2 * phaseS / cc\n\n    rms=0\n    for x=pointsPerCycle, smua.nvbuffer2.n do\n      v=\tsmua.nvbuffer1[x]\n      rms=rms + (v-mid)*(v-mid)\n    end\n    rms = math.sqrt(rms/cc)\n\n    phase = 0\n    cc=0\n    for c=1,numCycles-1 do\n\t\tx0=pointsPerCycle*c\n\t\tfor x=x0+1,x0+pointsPerCycle-2 do\n             if ( smua.nvbuffer1[x]<=mid and  smua.nvbuffer1[x+1]>mid) then\n\t\t\t\tphase =phase + (x-x0)/pointsPerCycle\n                cc=cc+1\n\t\t\t\tbreak\n\t\t\t end\n\t\tend\n\tend\n   \n   pointsPerCycle=math.floor(pointsPerCycle)\n   omega=frequency*2*math.pi\n   print(frequency, VLin, Vpp, phaseC/Vpp* math.sqrt(omega) *1565856180.88521 -57.2098793899397 , rms/Vrms, phaseC/Vpp, phaseS/Vpp,rms,2*math.pi* phase/cc)\n  \nend\n\n\n\n\nfunction Square_Waveform_Sweep(Vrms, numCycles, frequency, limitI)\n    reset()\n    local COMPLETE = \"{COMPLETE}\"\n    -- Generate the source values\n    local Vpp = Vrms * math.sqrt(2)\n    local sourceValues = {}\n    local pointsPerCycle = 7200 / frequency\n    local numDataPoints = pointsPerCycle * numCycles\n\n    for i = 1, numDataPoints do\n        if ((Vpp * math.sin(i * 2 * math.pi / pointsPerCycle)) < 0) then\n            sourceValues[i] = Vpp\n        else\n            sourceValues[i] = 0\n        end\n    end\n\n    -- Configure the SMU ranges\n    smua.reset()\n    smua.source.settling = smua.SETTLE_FAST_POLARITY\n    smua.source.autorangev = smua.AUTORANGE_OFF\n    smua.source.autorangei = smua.AUTORANGE_OFF\n    smua.source.rangev = Vpp\n    smua.source.delay = 0\n    smua.source.limiti = 1e-12\n\n    smua.measure.autorangev = smua.AUTORANGE_OFF\n    smua.measure.autorangei = smua.AUTORANGE_OFF\n    smua.measure.autozero = smua.AUTOZERO_OFF\n    smua.measure.delay = 0\n    smua.measure.delayfactor = 1\n    smua.measure.analogfilter = 0\n\n    -- Voltage will be measured on the same range as the source range\n    smua.measure.rangei = limitI\n    smua.measure.nplc = 0.001\n\n    -- Prepare the Reading Buffers\n    smua.nvbuffer1.clear()\n    smua.nvbuffer1.collecttimestamps = 1\n    smua.nvbuffer2.clear()\n    smua.nvbuffer2.collecttimestamps = 1\n\n    -- Configure the trigger model\n    -- ============================\n\n    -- Timer 1 controls the time between source points\n    trigger.timer[1].delay = (1 / 7200)\n    trigger.timer[1].passthrough = true\n    trigger.timer[1].stimulus = smua.trigger.ARMED_EVENT_ID\n    trigger.timer[1].count = numDataPoints - 1\n\n    -- Configure the SMU trigger model\n    smua.trigger.source.listv(sourceValues)\n    smua.trigger.source.limiti = limitI\n    smua.trigger.measure.action = smua.ENABLE\n    smua.trigger.measure.iv(smua.nvbuffer1, smua.nvbuffer2)\n    smua.trigger.endpulse.action = smua.SOURCE_HOLD\n    smua.trigger.endsweep.action = smua.SOURCE_IDLE\n    smua.trigger.count = numDataPoints\n    smua.trigger.arm.stimulus = 0\n    smua.trigger.source.stimulus = trigger.timer[1].EVENT_ID\n    smua.trigger.measure.stimulus = 0\n    smua.trigger.endpulse.stimulus = 0\n    smua.trigger.source.action = smua.ENABLE\n    -- Ready to begin the test\n\n    smua.source.output = smua.OUTPUT_ON\n    -- Start the trigger model execution\n    smua.trigger.initiate()\n    -- Wait until the sweep has completed\n    waitcomplete()\n    smua.source.output = smua.OUTPUT_OFF\n\n    -- Print the data back to the Console in tabular format\n    singleWave = {}\n    visits = {}\n    size1 = 0\n    for x = 1, smua.nvbuffer2.n do\n        local i = math.floor(x - math.floor(x / (pointsPerCycle)) * (pointsPerCycle))\n        v = smua.nvbuffer1[x]\n        if (math.abs(v) < 1e-3) then\n            if (singleWave[i] == nil) then\n                singleWave[i] = v\n                visits[i] = 1\n                if (size1 < i) then\n                    size1 = i\n                end\n            else\n                singleWave[i] = singleWave[i] + v\n                visits[i] = visits[i] + 1\n            end\n        end\n        --    print(smua.nvbuffer1.timestamps[x], smua.nvbuffer2[x], smua.nvbuffer1[x],i,singleWave[i])\n    end\n\n    \n    maxV = 0\n    maxI = 0\n    timeI = 0\n    for x = 1, size1 do\n        singleWave[x] = singleWave[x] / visits[x]\n        v = smua.nvbuffer2[x + pointsPerCycle]\n        if (v > maxV) then\n            maxV = v\n        end\n        if (singleWave[x] > maxI) then\n            maxI = singleWave[x]\n            timeI = x\n        end\n    end\n\n    pointsPerCycle = math.floor(pointsPerCycle)\n    timeEnd =0\n    for x = timeI, size1 - 1 do\n        --print(smua.nvbuffer1.timestamps[x] - smua.nvbuffer1.timestamps[timeI], smua.nvbuffer2[x + pointsPerCycle],            singleWave[x] / maxI)\n        i = singleWave[x] / maxI\n        if (i < .36) then\n            timeEnd = smua.nvbuffer1.timestamps[x] - smua.nvbuffer1.timestamps[timeI]\n            break\n        end\n    end\n    \n    print(frequency, 0, Vpp, timeEnd/4031000 , maxI/Vpp, timeEnd,0,maxI,timeEnd)\n\nend\n\nif (doCap==1) then \n    AC_Waveform_Sweep(.01,0, 15, 30,  10e-9,10)\n    AC_Waveform_Sweep(.01,0, 30, 60,  10e-9,5)\n    AC_Waveform_Sweep(.01,0, 100, 200,  10e-9,1)\n    AC_Waveform_Sweep(.01,0, 150, 300,  10e-9,1)\n\n    AC_Waveform_Sweep(.01,-.1, 200, 400,  10e-9,1)\n    AC_Waveform_Sweep(.01,-.05, 200, 400,  10e-9,1)\n    AC_Waveform_Sweep(.01,0.0, 200, 400,  10e-9,1)\n    AC_Waveform_Sweep(.01,0.05, 200, 400,  10e-9,1)\n    AC_Waveform_Sweep(.01,0.1, 200, 400,  10e-9,1)\n\n    Square_Waveform_Sweep(.01, 40, 80,  10e-9)\nelse \n    for c=1,10 do\n        print(0, 0, 0, 0 , 0, 0,0,0,0)\n    end\nend\n\nprint(\"{COMPLETE}\")\n\n\n", 8 "CurrentRange":dbl=1e-10, 9 "Source Measure Unit Channel (0: Channel A)":i32, 10 "Waveform":waveform(dbl), 11 "VISA Refnum in":refnum<visa-resource-name>) -> (1 "appended array":dbl[][](array[numeric]), 3 "InfoCluster":T1)   [LabVIEW 2020]
uses:
  CapacitanceRecord.ctl
  CapacitanceInfos.ctl
  Keithley 2600 Series/Keithley 2600 Series.lvlib
panel:
  out "CapacitanceRecords":T2[](array[typedef])
  out "Device":dbl[][](array[numeric])=[[0.0, 0.099997, 0.199996, 0.299996, 0.399996, 0.499997, 0.599996, 0.699997, 0.799997, 0.899996, 0.0, 0.099997, 0.199996, 0.299996, 0.399996, 0.499997, 0.599996, 0.699997, 0.799997, 0.899996, 0.999996, 1.099997, 1.199997, 1.299996, 1.399996, 1.499996, 1.599996, 1.699996, 1.799996, 1.899996, 0.999996, 1.099997, 1.199997, 1.299996, 1.399996, 1.499996, 1.599996, 1.699996, 1.799996, 1.899996, 1.999996, 2.099996, 2.199997, 2.299996, 2.399996, 2.499997, 2.599997, 2.699996, 2.799996, 2.899997, 2.999996, 1.999996, 2.099996, 2.199997, 2.299996, 2.399996, 2.499997, 2.599997, 2.699996, 2.799996, 2.899997, 2.999996, 3.099996, 3.199996, 3.299997, 3.399996, 3.499997, 3.599996, 3.699996, 3.799997, 3.899996, 3.999997, 3.099996, 3.199996, 3.299997, 3.399996, 3.499997, 3.599996, 3.699996, 3.799997, 3.899996, 3.999997, 4.099997, 4.199996, 4.299997, 4.399996, 4.499997, 4.599997, 4.699996, 4.799996, 4.899996, 5.000106, 4.099997, 4.199996, 4.299997, 4.399996, 4.499997, 4.599997, 4.699996, 4.799996, 4.899996, 5.000106, 5.099996, 5.199996, 5.299997, 5.399996, 5.499996, 5.599996, 5.699996, 5.799997, 5.899997, 5.999996, 5.099996, 5.199996, 5.299997, 5.399996, 5.499996, 5.599996, 5.699996, 5.799997, 5.899997, 5.999996, 6.099997, 6.199997, 6.300001, 6.399997, 6.499996, 6.599996, 6.699996, 6.799996, 6.899996, 6.999996, 6.099997, 6.199997, 6.300001, 6.399997, 6.499996, 6.599996, 6.699996, 6.799996, 6.899996, 6.999996, 7.099996, 7.199997, 7.299996, 7.399996, 7.499996, 7.599996, 7.699996, 7.799997, 7.899996, 7.999996, 7.099996, 7.199997, 7.299996, 7.399996, 7.499996, 7.599996, 7.699996, 7.799997, 7.899996, 7.999996, 8.099997, 8.199997, 8.299997, 8.399996, 8.499996, 8.599996, 8.699996, 8.799996, 8.899997, 8.999996, 8.099997, 8.199997, 8.299997, 8.399996, 8.499996, 8.599996, 8.699996, 8.799996, 8.899997, 8.999996, 9.099996, 9.199996, 9.299997, 9.399997, 9.499996, 9.599996, 9.699996, 9.799997, 9.900105, 9.999996, 9.099996, 9.199996, 9.299997, 9.399997, 9.499996, 9.599996, 9.699996, 9.799997, 9.900105, 9.999996, 10.1, 10.2, 10.3, 10.4, 10.5, 10.6, 10.7, 10.8, 10.9, 11.0, 10.1, 10.2, 10.3, 10.4, 10.5, 10.6, 10.7, 10.8, 10.9, 11.0, 11.1, 11.2, 11.3, 11.4, 11.5, 11.6, 11.7, 11.8, 11.9, 12.0, 11.1, 11.2, 11.3, 11.4, 11.5, 11.6, 11.7, 11.8, 11.9, 12.0, 12.1, 12.2, 12.3, 12.4, 12.5, 12.6, 12.7, 12.8, 12.9, 13.0, 12.1, 12.2, 12.3, 12.4, 12.5, 12.6, 12.7, 12.8, 12.9, 13.0, 13.1, 13.1, 13.2, 13.3, 13.4, 13.5, 13.6, 13.7, 13.8, 13.9, 14.0, 14.1, 13.2, 13.3, 13.4, 13.5, 13.6, 13.7, 13.8, 13.9, 14.0, 14.1, 14.2, 14.3, 14.4, 14.5, 14.6, 14.7, 14.8, 14.9, 15.0001, 15.1, 14.2, 14.3, 14.4, 14.5, 14.6, 14.7, 14.8, 14.9, 15.0001, 15.1, 15.2, 15.3, 15.4, 15.5, 15.6, 15.7, 15.8, 15.9, 16.0, 16.1, 15.2, 15.3, 15.4, 15.5, 15.6, 15.7, 15.8, 15.9, 16.0, 16.1, 16.2, 16.3, 16.4, 16.5, 16.6, 16.7, 16.8, 16.9, 17.0, 17.1, 16.2, 16.3, 16.4, 16.5, 16.6, 16.7, 16.8, 16.9, 17.0, 17.1, 17.2, 17.3, 17.4, 17.5, 17.6, 17.7, 17.8, 17.9, 18.0, 18.1, 17.2, 17.3, 17.4, 17.5, 17.6, 17.7, 17.8, 17.9, 18.0, 18.1, 18.2, 18.3, 18.4, 18.5, 18.6, 18.7, 18.8, 18.9, 19.0, 19.1, 18.2, 18.3, 18.4, 18.5, 18.6, 18.7, 18.8, 18.9, 19.0, 19.1, 19.2, 19.3, 19.4, 19.5, 19.6, 19.7, 19.8, 19.90011, 19.2, 19.3, 19.4, 19.5, 19.6, 19.7, 19.8, 19.90011], [0.004, 0.008, 0.012, 0.016, 0.02, 0.024, 0.028, 0.032, 0.036, 0.04, 0.004, 0.008, 0.012, 0.016, 0.02, 0.024, 0.028, 0.032, 0.036, 0.04, 0.044, 0.048, 0.052, 0.056, 0.06, 0.064, 0.068, 0.072, 0.076, 0.08, 0.044, 0.048, 0.052, 0.056, 0.06, 0.064, 0.068, 0.072, 0.076, 0.08, 0.084, 0.088, 0.092, 0.096, 0.1, 0.096, 0.092, 0.088, 0.084, 0.08, 0.076, 0.084, 0.088, 0.092, 0.096, 0.1, 0.096, 0.092, 0.088, 0.084, 0.08, 0.076, 0.072, 0.068, 0.064, 0.06, 0.056, 0.052, 0.048, 0.044, 0.04, 0.036, 0.072, 0.068, 0.064, 0.06, 0.056, 0.052, 0.048, 0.044, 0.04, 0.036, 0.032, 0.028, 0.024, 0.02, 0.016, 0.012, 0.008, 0.004, 0.0, -0.004, 0.032, 0.028, 0.024, 0.02, 0.016, 0.012, 0.008, 0.004, 0.0, -0.004, -0.008, -0.012, -0.016, -0.02, -0.024, -0.028, -0.032, -0.036, -0.04, -0.044, -0.008, -0.012, -0.016, -0.02, -0.024, -0.028, -0.032, -0.036, -0.04, -0.044, -0.048, -0.052, -0.056, -0.06, -0.064, -0.068, -0.072, -0.076, -0.08, -0.084, -0.048, -0.052, -0.056, -0.06, -0.064, -0.068, -0.072, -0.076, -0.08, -0.084, -0.088, -0.092, -0.096, -0.1, -0.096, -0.092, -0.088, -0.084, -0.08, -0.076, -0.088, -0.092, -0.096, -0.1, -0.096, -0.092, -0.088, -0.084, -0.08, -0.076, -0.072, -0.068, -0.064, -0.06, -0.056, -0.052, -0.048, -0.044, -0.04, -0.036, -0.072, -0.068, -0.064, -0.06, -0.056, -0.052, -0.048, -0.044, -0.04, -0.036, -0.032, -0.028, -0.024, -0.02, -0.016, -0.012, -0.008, -0.004, 0.0, 0.004, -0.032, -0.028, -0.024, -0.02, -0.016, -0.012, -0.008, -0.004, 0.0, 0.004, 0.008, 0.012, 0.016, 0.02, 0.024, 0.028, 0.032, 0.036, 0.04, 0.044, 0.008, 0.012, 0.016, 0.02, 0.024, 0.028, 0.032, 0.036, 0.04, 0.044, 0.048, 0.052, 0.056, 0.06, 0.064, 0.068, 0.072, 0.076, 0.08, 0.084, 0.048, 0.052, 0.056, 0.06, 0.064, 0.068, 0.072, 0.076, 0.08, 0.084, 0.088, 0.092, 0.096, 0.1, 0.096, 0.092, 0.088, 0.084, 0.08, 0.076, 0.088, 0.092, 0.096, 0.1, 0.096, 0.092, 0.088, 0.084, 0.08, 0.076, 0.072, 0.072, 0.068, 0.064, 0.06, 0.056, 0.052, 0.048, 0.044, 0.04, 0.036, 0.032, 0.068, 0.064, 0.06, 0.056, 0.052, 0.048, 0.044, 0.04, 0.036, 0.032, 0.028, 0.024, 0.02, 0.016, 0.012, 0.008, 0.004, 0.0, -0.004, -0.008, 0.028, 0.024, 0.02, 0.016, 0.012, 0.008, 0.004, 0.0, -0.004, -0.008, -0.012, -0.016, -0.02, -0.024, -0.028, -0.032, -0.036, -0.04, -0.044, -0.048, -0.012, -0.016, -0.02, -0.024, -0.028, -0.032, -0.036, -0.04, -0.044, -0.048, -0.052, -0.056, -0.06, -0.064, -0.068, -0.072, -0.076, -0.08, -0.084, -0.088, -0.052, -0.056, -0.06, -0.064, -0.068, -0.072, -0.076, -0.08, -0.084, -0.088, -0.092, -0.096, -0.1, -0.096, -0.092, -0.088, -0.084, -0.08, -0.076, -0.072, -0.092, -0.096, -0.1, -0.096, -0.092, -0.088, -0.084, -0.08, -0.076, -0.072, -0.068, -0.064, -0.06, -0.056, -0.052, -0.048, -0.044, -0.04, -0.036, -0.032, -0.068, -0.064, -0.06, -0.056, -0.052, -0.048, -0.044, -0.04, -0.036, -0.032, -0.028, -0.024, -0.02, -0.016, -0.012, -0.008, -0.004, 0.0, -0.028, -0.024, -0.02, -0.016, -0.012, -0.008, -0.004, 0.0], [0.004012108, 0.008024216, 0.01200104, 0.01601458, 0.02002883, 0.02400613, 0.02802062, 0.0319972, 0.03600836, 0.04002452, 0.0440011, 0.04801679, 0.05203104, 0.05601096, 0.06002402, 0.06400466, 0.06801891, 0.07203341, 0.07601213, 0.08002782, 0.08400989, 0.08802176, 0.09204006, 0.09601855, 0.1000333, 0.09601688, 0.09203887, 0.08802152, 0.08400989, 0.08003378, 0.07601571, 0.07203484, 0.06802511, 0.06401062, 0.06003165, 0.05601764, 0.05203867, 0.04802275, 0.04400706, 0.04003, 0.03601575, 0.03200626, 0.02802396, 0.02401495, 0.02003837, 0.01601982, 0.01200485, 0.008026361, 0.004018784, 3.957748e-05, -0.003931522, -0.00793457, -0.01190996, -0.01592636, -0.01994705, -0.02392316, -0.02793789, -0.03195095, -0.0359273, -0.03994632, -0.04392123, -0.04793477, -0.05194736, -0.05592632, -0.05994105, -0.06395578, -0.06793571, -0.07194591, -0.07592487, -0.07993889, -0.08395553, -0.08793473, -0.09195065, -0.09596539, -0.09994173, -0.09596539, -0.09195185, -0.08793402, -0.08395767, -0.07994437, -0.07593036, -0.0719502, -0.06793904, -0.06396365, -0.05994511, -0.05593252, -0.05195069, -0.04793167, -0.04392576, -0.03994441, -0.0359323, -0.03195429, -0.02793765, -0.02392602, -0.01994729, -0.01593328, -0.01191473, -0.007936478, -0.003926039, 4.601479e-05, 0.004010439, 0.008024931, 0.01199889, 0.01601291, 0.02003217, 0.02401352, 0.02802873, 0.03200412, 0.03601956, 0.04002929, 0.04400897, 0.04802442, 0.05203891, 0.05601859, 0.06003046, 0.06400704, 0.06801963, 0.07203436, 0.07601428, 0.08002687, 0.08400512, 0.08802056, 0.09204149, 0.0960176, 0.1000292, 0.09601521, 0.09204412, 0.08802152, 0.08401251, 0.08003378, 0.07601666, 0.07204151, 0.06802106, 0.06400704, 0.06003046, 0.05601192, 0.05203247, 0.04801679, 0.04400253, 0.04002523, 0.03601003, 0.0319972, 0.02802181, 0.02400851, 0.02003407, 0.0160141, 0.01199675, 0.008023262, 0.004011631, 3.194809e-05, -0.003937483, -0.007942438, -0.01191759, -0.01592827, -0.01994705, -0.02392673, -0.02793503, -0.03195024, -0.03593087, -0.03994489, -0.04392171, -0.04793072, -0.05195022, -0.05592752, -0.0599401, -0.06395555, -0.06792974, -0.07194424, -0.07592344, -0.0799365, -0.08394909, -0.08793044, -0.0919466, -0.09596252, -0.09994292, -0.09596872, -0.09195304, -0.08793187, -0.0839572, -0.07994318, -0.07593107, -0.07194948, -0.06793761, -0.06396294, -0.05994534, -0.05592918, -0.05194783, -0.04794264, -0.04392028, -0.03993964, -0.03592658, -0.03195238, -0.02793765, -0.02392507, -0.01995111, -0.01593399, -0.01192093, -0.007943153, -0.003931284, 4.36306e-05, 0.0, 0.0, 0.0, 0.0, 0.0, 0.0, 0.0, 0.0, 0.0, 0.0, 0.0, 0.0, 0.0, 0.0, 0.0, 0.0, 0.0, 0.0, 0.0, 0.0, 0.0, 0.0, 0.0, 0.0, 0.0, 0.0, 0.0, 0.0, 0.0, 0.0, 0.0, 0.0, 0.0, 0.0, 0.0, 0.0, 0.0, 0.0, 0.0, 0.0, 0.0, 0.0, 0.0, 0.0, 0.0, 0.0, 0.0, 0.0, 0.0, 0.0, 0.0, 0.0, 0.0, 0.0, 0.0, 0.0, 0.0, 0.0, 0.0, 0.0, 0.0, 0.0, 0.0, 0.0, 0.0, 0.0, 0.0, 0.0, 0.0, 0.0, 0.0, 0.0, 0.0, 0.0, 0.0, 0.0, 0.0, 0.0, 0.0, 0.0, 0.0, 0.0, 0.0, 0.0, 0.0, 0.0, 0.0, 0.0, 0.0, 0.0, 0.0, 0.0, 0.0, 0.0, 0.0, 0.0, 0.0, 0.0, 0.0, 0.0, 0.0, 0.0, 0.0, 0.0, 0.0, 0.0, 0.0, 0.0, 0.0, 0.0, 0.0, 0.0, 0.0, 0.0, 0.0, 0.0, 0.0, 0.0, 0.0, 0.0, 0.0, 0.0, 0.0, 0.0, 0.0, 0.0, 0.0, 0.0, 0.0, 0.0, 0.0, 0.0, 0.0, 0.0, 0.0, 0.0, 0.0, 0.0, 0.0, 0.0, 0.0, 0.0, 0.0, 0.0, 0.0, 0.0, 0.0, 0.0, 0.0, 0.0, 0.0, 0.0, 0.0, 0.0, 0.0, 0.0, 0.0, 0.0, 0.0, 0.0, 0.0, 0.0, 0.0, 0.0, 0.0, 0.0, 0.0, 0.0, 0.0, 0.0, 0.0, 0.0, 0.0, 0.0, 0.0, 0.0, 0.0, 0.0, 0.0, 0.0, 0.0, 0.0, 0.0, 0.0, 0.0, 0.0, 0.0, 0.0, 0.0, 0.0, 0.0, 0.0, 0.0, 0.0, 0.0, 0.0, 0.0, 0.0, 0.0, 0.0], [4.876375e-13, 8.405447e-13, 1.041794e-12, 1.124167e-12, 1.170063e-12, 1.180363e-12, 1.183665e-12, 1.205146e-12, 1.251078e-12, 1.208818e-12, 1.196444e-12, 1.235938e-12, 1.178539e-12, 1.208818e-12, 1.19698e-12, 1.231945e-12, 1.229155e-12, 1.189446e-12, 1.236415e-12, 1.199806e-12, 1.146781e-12, 1.230025e-12, 1.219225e-12, 1.240659e-12, 1.235735e-12, -9.934902e-14, -6.992459e-13, -1.09061e-12, -1.198101e-12, -1.301944e-12, -1.323438e-12, -1.324773e-12, -1.261115e-12, -1.266289e-12, -1.349556e-12, -1.353908e-12, -1.372743e-12, -1.393998e-12, -1.407564e-12, -1.390636e-12, -1.3937e-12, -1.39513e-12, -1.341021e-12, -1.334751e-12, -1.329553e-12, -1.382935e-12, -1.465642e-12, -1.445627e-12, -1.427853e-12, -1.445568e-12, -1.310861e-12, -1.378262e-12, -1.38613e-12, -1.476145e-12, -1.421046e-12, -1.50212e-12, -1.475501e-12, -1.468349e-12, -1.43584e-12, -1.38098e-12, -1.364648e-12, -1.414478e-12, -1.467621e-12, -1.457799e-12, -1.511776e-12, -1.457047e-12, -1.472986e-12, -1.465058e-12, -1.470017e-12, -1.449299e-12, -1.483786e-12, -1.433086e-12, -1.415682e-12, -1.443815e-12, -1.382887e-12, -2.35796e-14, 4.857421e-13, 7.995486e-13, 8.286357e-13, 1.046395e-12, 1.058543e-12, 1.10774e-12, 1.014256e-12, 1.110172e-12, 1.107299e-12, 1.152408e-12, 1.177096e-12, 1.099634e-12, 1.013386e-12, 1.027525e-12, 9.33969e-13, 9.427667e-13, 1.007175e-12, 1.04382e-12, 1.113117e-12, 1.106226e-12, 1.08093e-12, 1.09967e-12, 1.149261e-12, 1.07007e-12, 1.20064e-12, 1.104999e-12, 1.004756e-12, 1.033092e-12, 1.066244e-12, 1.089573e-12, 1.147914e-12, 1.204836e-12, 1.188779e-12, 1.286149e-12, 1.25159e-12, 1.136637e-12, 1.113093e-12, 1.14038e-12, 1.287889e-12, 1.228535e-12, 1.111662e-12, 1.184595e-12, 1.079833e-12, 1.099265e-12, 1.151586e-12, 1.186442e-12, 1.185751e-12, 1.190615e-12, 1.187813e-12, -8.373261e-14, -7.273317e-13, -1.092684e-12, -1.197386e-12, -1.276159e-12, -1.419008e-12, -1.401079e-12, -1.389229e-12, -1.510131e-12, -1.403821e-12, -1.414502e-12, -1.405585e-12, -1.397002e-12, -1.436079e-12, -1.32556e-12, -1.342237e-12, -1.391172e-12, -1.414716e-12, -1.417804e-12, -1.446748e-12, -1.480424e-12, -1.397955e-12, -1.412237e-12, -1.420128e-12, -1.371849e-12, -1.297367e-12, -1.3973e-12, -1.367521e-12, -1.469433e-12, -1.385069e-12, -1.438558e-12, -1.454413e-12, -1.419246e-12, -1.437104e-12, -1.439106e-12, -1.477444e-12, -1.434636e-12, -1.511836e-12, -1.413178e-12, -1.417887e-12, -1.464427e-12, -1.446223e-12, -1.510513e-12, -1.421475e-12, -1.431835e-12, -1.426148e-12, -1.296699e-12, -1.461732e-12, -1.408112e-12, -1.400995e-12, -1.352072e-13, 4.454851e-13, 7.381081e-13, 9.427428e-13, 1.014519e-12, 1.077449e-12, 1.152933e-12, 1.153064e-12, 1.096571e-12, 1.185477e-12, 1.118922e-12, 1.124501e-12, 1.121414e-12, 1.092613e-12, 1.154149e-12, 1.070058e-12, 1.105118e-12, 1.156211e-12, 1.252687e-12, 1.177442e-12, 1.202261e-12, 1.197708e-12, 1.185524e-12, 1.162577e-12, 1.069427e-12, 0.0, 0.0, 0.0, 0.0, 0.0, 0.0, 0.0, 0.0, 0.0, 0.0, 0.0, 0.0, 0.0, 0.0, 0.0, 0.0, 0.0, 0.0, 0.0, 0.0, 0.0, 0.0, 0.0, 0.0, 0.0, 0.0, 0.0, 0.0, 0.0, 0.0, 0.0, 0.0, 0.0, 0.0, 0.0, 0.0, 0.0, 0.0, 0.0, 0.0, 0.0, 0.0, 0.0, 0.0, 0.0, 0.0, 0.0, 0.0, 0.0, 0.0, 0.0, 0.0, 0.0, 0.0, 0.0, 0.0, 0.0, 0.0, 0.0, 0.0, 0.0, 0.0, 0.0, 0.0, 0.0, 0.0, 0.0, 0.0, 0.0, 0.0, 0.0, 0.0, 0.0, 0.0, 0.0, 0.0, 0.0, 0.0, 0.0, 0.0, 0.0, 0.0, 0.0, 0.0, 0.0, 0.0, 0.0, 0.0, 0.0, 0.0, 0.0, 0.0, 0.0, 0.0, 0.0, 0.0, 0.0, 0.0, 0.0, 0.0, 0.0, 0.0, 0.0, 0.0, 0.0, 0.0, 0.0, 0.0, 0.0, 0.0, 0.0, 0.0, 0.0, 0.0, 0.0, 0.0, 0.0, 0.0, 0.0, 0.0, 0.0, 0.0, 0.0, 0.0, 0.0, 0.0, 0.0, 0.0, 0.0, 0.0, 0.0, 0.0, 0.0, 0.0, 0.0, 0.0, 0.0, 0.0, 0.0, 0.0, 0.0, 0.0, 0.0, 0.0, 0.0, 0.0, 0.0, 0.0, 0.0, 0.0, 0.0, 0.0, 0.0, 0.0, 0.0, 0.0, 0.0, 0.0, 0.0, 0.0, 0.0, 0.0, 0.0, 0.0, 0.0, 0.0, 0.0, 0.0, 0.0, 0.0, 0.0, 0.0, 0.0, 0.0, 0.0, 0.0, 0.0, 0.0, 0.0, 0.0, 0.0, 0.0, 0.0, 0.0, 0.0, 0.0, 0.0, 0.0, 0.0, 0.0, 0.0, 0.0, 0.0, 0.0, 0.0, 0.0, 0.0, 0.0, 0.0, 0.0]]
  out "XY Graph 2":cluster{dbl[], dbl[]}[](graph)
  out "Waveform Graph":waveform(dbl)(graph)
  out "XY Graph":T3(graph)
  out "error out":errorcluster
  in  "Script Variable (myScript)":string="myScript"
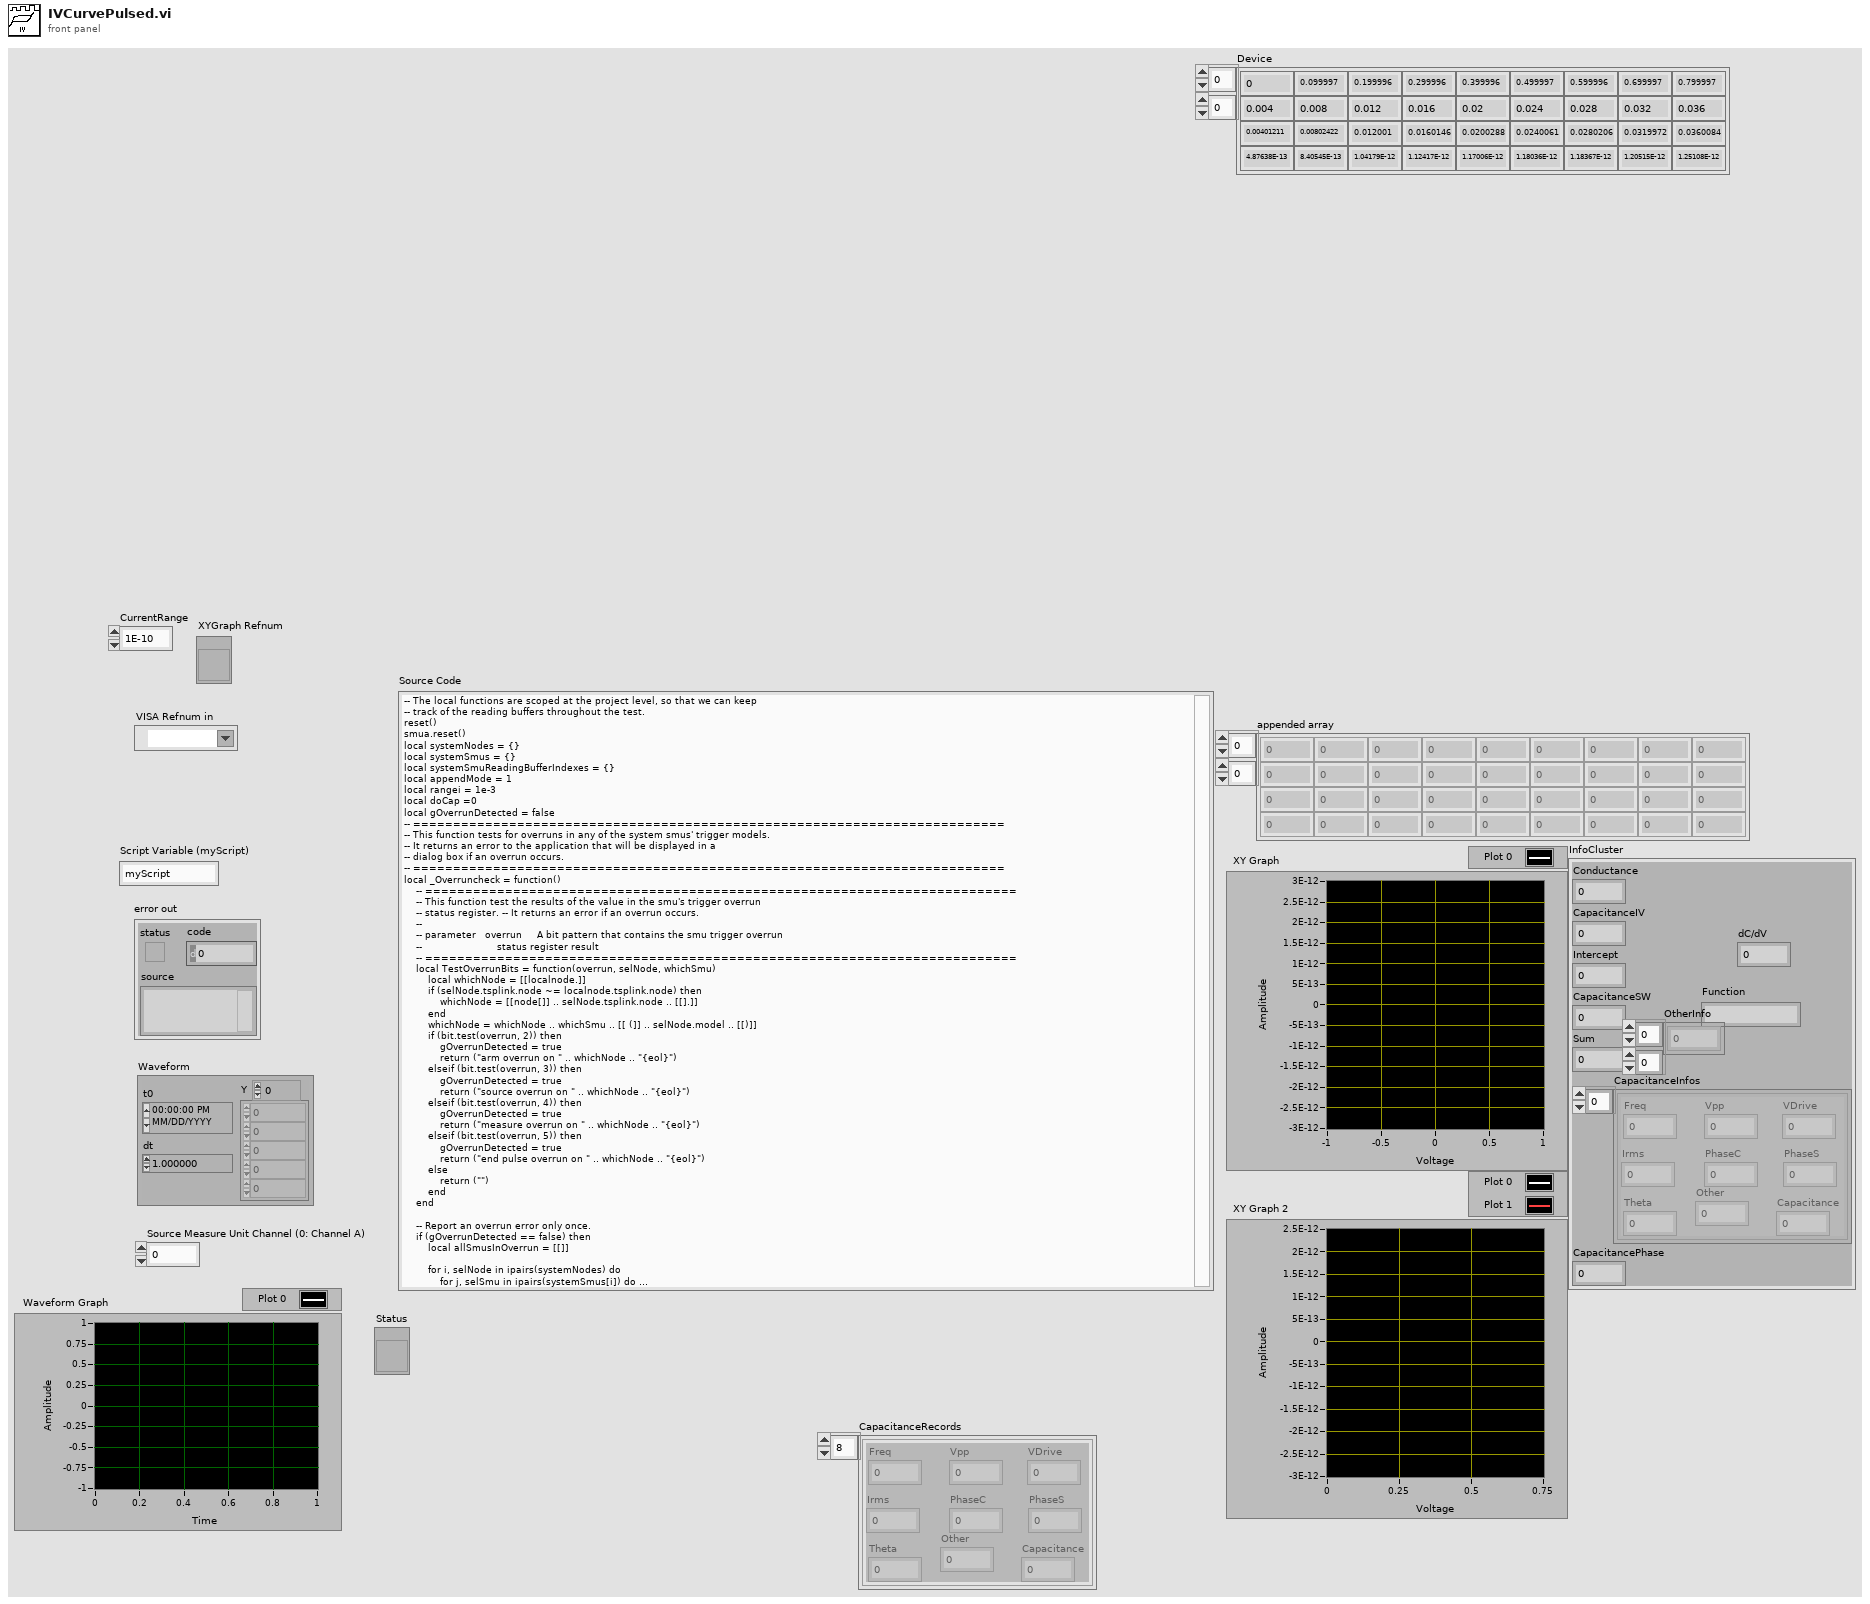
[diagram p1: front panel]
types:
  T1 = typedef "CapacitanceInfos.ctl" = cluster{"Conductance":dbl, "CapacitanceIV":dbl, "Intercept":dbl, "CapacitanceSW":dbl, "Sum":dbl, "CapacitanceInfos":T2[], "CapacitancePhase":dbl, "dC/dV":dbl, "Function":string, "OtherInfo":dbl[][]}
  T2 = typedef "CapacitanceRecord.ctl" = cluster{"Freq":dbl, "Vpp":dbl, "PhaseS":dbl, "Irms":dbl, "PhaseC":dbl, "Theta":dbl, "VDrive":dbl, "Capacitance":dbl, "Other":dbl}
  T3 = cluster{"array type (2D Dbl)":dbl[], "array type (2D Dbl)":dbl[]}
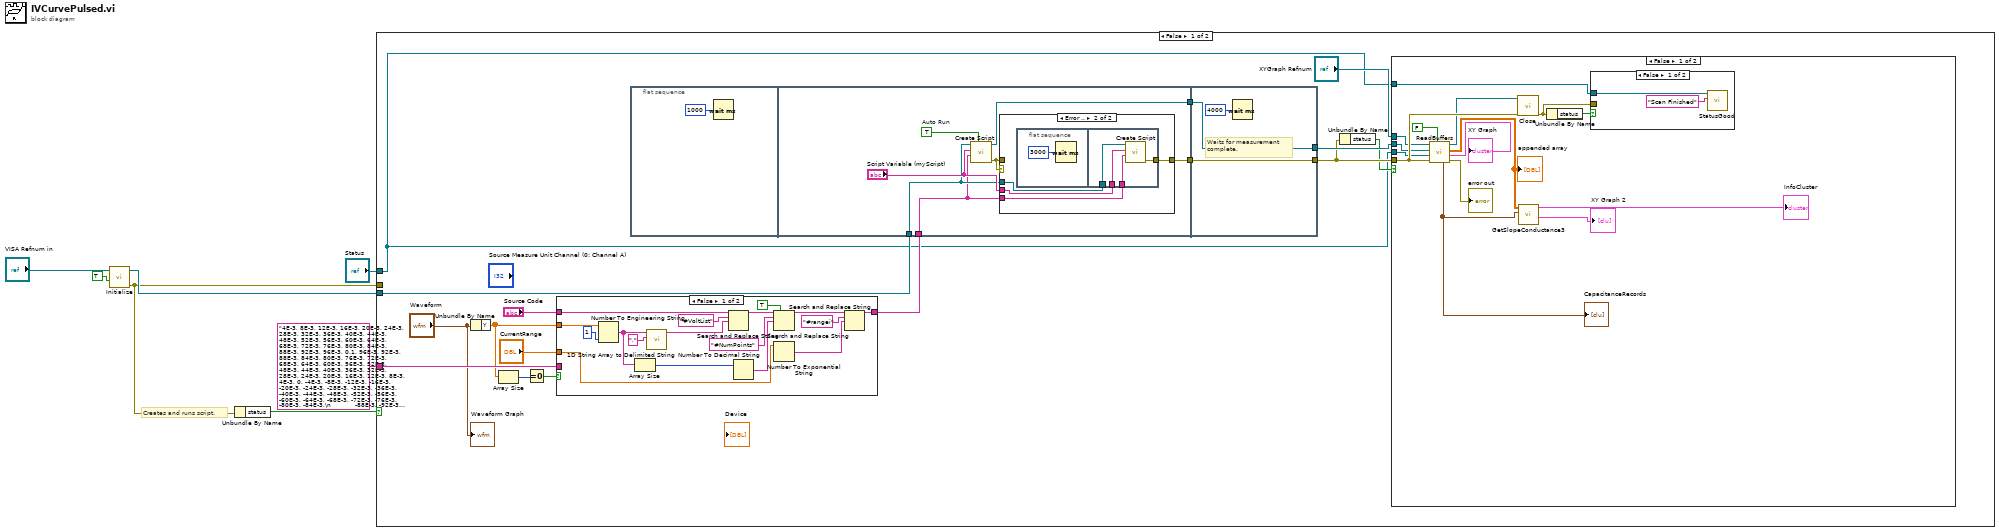
[diagram p0: block diagram]
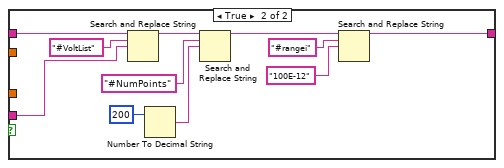
[diagram p2: hidden frame]
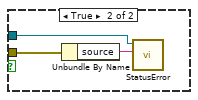
[diagram p3: hidden frame]
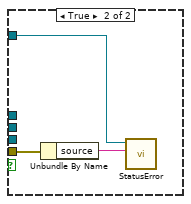
[diagram p4: hidden frame]
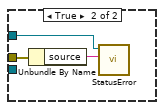
[diagram p6: hidden frame]
diagram:
  # "Creates and runs script."
  n1 = call "Initialize.vi"("Reset (True)"=TRUE, "VISA resource name"="VISA Refnum in") -> ("error out"=w1:errorcluster, "VISA resource name out"=w6:refnum<visa-resource-name>)  [unwired: 8 in]
  n2 = Unbundle By Name(w1) -> ("status"=w4:bool)
  n3 = case shown="False" w4 {
    tunnel: w6 -> [w10 _]
    tunnel: "4E-3, 8E-3, 12E-3, 16E-3, 20E-3, 24E-3, 28E-3, 32E-3, 36E-3, 40E-3, 44E-3, 48E-3, 52E-3, 56E-3, 60E-3, 64E-3, 68E-3, 72E-3, 76E-3, 80E-3, 84E-3, 88E-3, 92E-3, 96E-3, 0.1, 96E-3, 92E-3, 88E-3, 84E-3, 80E-3, 76E-3, 72E-3, 68E-3, 64E-3, 60E-3, 56E-3, 52E-3, 48E-3, 44E-3, 40E-3, 36E-3, 32E-3, 28E-3, 24E-3, 20E-3, 16E-3, 12E-3, 8E-3, 4E-3, 0, -4E-3, -8E-3, -12E-3, -16E-3, -20E-3, -24E-3, -28E-3, -32E-3, -36E-3, -40E-3, -44E-3, -48E-3, -52E-3, -56E-3, -60E-3, -64E-3, -68E-3, -72E-3, -76E-3, -80E-3, -84E-3,\n            -88E-3, -92E-3, -96E-3, -0.1, -96E-3, -92E-3, -88E-3, -84E-3, -80E-3, -76E-3, -72E-3, -68E-3, -64E-3, -60E-3, -56E-3, -52E-3, -48E-3, -44E-3, -40E-3, -36E-3, -32E-3, -28E-3, -24E-3, -20E-3, -16E-3, -12E-3, -8E-3, -4E-3, 0, 4E-3, 8E-3, 12E-3, 16E-3, 20E-3, 24E-3, 28E-3, 32E-3, 36E-3, 40E-3, 44E-3, 48E-3, 52E-3, 56E-3, 60E-3, 64E-3, 68E-3, 72E-3, 76E-3, 80E-3, 84E-3, 88E-3, 92E-3, 96E-3, 0.1, 96E-3, 92E-3, 88E-3, 84E-3, 80E-3, 76E-3, 72E-3, 68E-3, 64E-3, 60E-3, 56E-3, 52E-3, 48E-3, 44E-3, 40E-3, 36E-3,\n        32E-3, 28E-3, 24E-3, 20E-3, 16E-3, 12E-3, 8E-3, 4E-3, 0, -4E-3, -8E-3, -12E-3, -16E-3, -20E-3, -24E-3, -28E-3, -32E-3, -36E-3, -40E-3, -44E-3, -48E-3, -52E-3, -56E-3, -60E-3, -64E-3, -68E-3, -72E-3, -76E-3, -80E-3, -84E-3, -88E-3, -92E-3, -96E-3, -0.1, -96E-3, -92E-3, -88E-3, -84E-3, -80E-3, -76E-3, -72E-3, -68E-3, -64E-3, -60E-3, -56E-3, -52E-3, -48E-3, -44E-3, -40E-3, -36E-3, -32E-3, -28E-3, -24E-3, -20E-3, -16E-3, -12E-3, -8E-3, -4E-3, 0" -> [w18 _]
    tunnel: "Status" -> [w8 w98]
    tunnel: w1 -> [_ w97]
    frame False {
      n4 = Unbundle By Name("Waveform") -> ("Y"=w11:dbl[])
      n5 = Array Size(array=w11) -> (size(s)=w14:i32)
      n6 = Equal To 0?(x=w14) -> (x = 0?=w13:bool)
      n7 = case shown="False" w13 {
        tunnel: w18 -> [_ w45]
        tunnel: [w27 w41] -> w17
        tunnel: "Source Code" -> [w30 w46]
        tunnel: w11 -> [w34 _]
        tunnel: "CurrentRange" -> [w25 _]
        frame False {
          n8 = Number To Engineering String(2:i16 1 ("precision (6)"), 4:w34) -> (0:w38:string[])  [unwired: 2 in]
          n9 = Array Size(array=w38) -> (size(s)=w39:i32)
          n10 = call <vilib>:"1D String Array to Delimited String.vi"("delimiter"=",", "string array"=w38) -> ("delimited string"=w36:string)  [unwired: 9 in]
          n11 = Search and Replace String(input string=w30, search string="#VoltList", replace string=w36) -> (result string=w37:string)  [unwired: 5 in, 3 out]
          n12 = Number To Decimal String(number=w39) -> (decimal integer string=w40:string)  [unwired: 1 in]
          n13 = Search and Replace String(replace all?=TRUE ("replace all? (F)"), input string=w37, search string="#NumPoints", replace string=w40) -> (result string=w28:string)  [unwired: 4 in, 3 out]
          n14 = Number To Exponential String(number=w25) -> (E-format string=w26:string)  [unwired: 3 in]
          n15 = Search and Replace String(input string=w28, search string="#rangei", replace string=w26) -> (result string=w27:string)  [unwired: 5 in, 3 out]
        }
        frame True {
          n16 = Search and Replace String(input string=w46, search string="#VoltList", replace string=w45) -> (result string=w51:string)  [unwired: 5 in, 3 out]
          n17 = Number To Decimal String(number=200) -> (decimal integer string=w49:string)  [unwired: 1 in]
          n18 = Search and Replace String(input string=w51, search string="#NumPoints", replace string=w49) -> (result string=w42:string)  [unwired: 5 in, 3 out]
          n19 = Search and Replace String(input string=w42, search string="#rangei", replace string="100E-12") -> (result string=w41:string)  [unwired: 5 in, 3 out]
        }
      }
      n20 = flat-sequence {
        tunnel: [w77] -> w23
        tunnel: [w82] -> w22
        tunnel: w17 -> [w78]
        tunnel: w10 -> [w79]
        tunnel: w23 -> [w95]
        tunnel: w22 -> [w94]
        tunnel: [w95] -> w20
        tunnel: [w94] -> w21
        frame #0 {
          n21 = Wait (ms)(milliseconds to wait=u32 1000) -> ()  [unwired: 1 out]
        }
        frame #1 {
          w81 = TRUE  # Auto Run
          n22 = call "Create Script.vi"("Auto Run (F: Disable)"=w81, "Source Code"=w78, "Script Variable"="Script Variable (myScript)", "VISA resource name"=w79) -> ("error out"=w76:errorcluster, "VISA resource name out"=w82:refnum<visa-resource-name>)  [unwired: 6 in]
          n23 = case shown="Error .." w76 {
            tunnel: "Script Variable (myScript)" -> [_ w87]
            tunnel: w79 -> [_ w86]
            tunnel: w78 -> [_ w85]
            tunnel: [w83 w84] -> w77
            tunnel: w76 -> [w83 _]
            frame No Error {
            }
            frame Error {
              n24 = flat-sequence {
                tunnel: w87 -> [w92]
                tunnel: w86 -> [w91]
                tunnel: w85 -> [w90]
                tunnel: [w89] -> w84
                frame #0 {
                  n25 = Wait (ms)(milliseconds to wait=u32 3000) -> ()  [unwired: 1 out]
                }
                frame #1 {
                  n26 = call "Create Script.vi"("Source Code"=w90, "Script Variable"=w92, "VISA resource name"=w91) -> ("error out"=w89:errorcluster)  [unwired: 7 in, 1 out]
                }
              }
            }
          }
        }
        frame #2 {
          # "Waits for measurement complete."
          n27 = Wait (ms)(milliseconds to wait=4000) -> ()  [unwired: 1 out]
        }
      }
      n28 = Unbundle By Name(w20) -> ("status"=w19:bool)
      n29 = case shown="False" w19 {
        tunnel: w20 -> [w66 w72]
        tunnel: w21 -> [w65 _]
        tunnel: "XYGraph Refnum" -> [w62 _]
        tunnel: w8 -> [w58 w73]
        tunnel: w8 -> [w57 _]
        frame False {
          n30 = call "ReadBuffers.vi"("CheckCap"=FALSE, "error in (no error)"=w66, "Status"=w57, "VISA resource name in"=w65, "XYGraph in"=w62) -> ("error out"=→"error out":errorcluster, "Cluster"=→"XY Graph":T3, "Array"=w55:dbl[][], "VISA Refnum out"=w64:refnum<visa-resource-name>, "CapacitanceRecords"=w52:T2[])  [unwired: 2 in]
          "appended array" <- w55
          "CapacitanceRecords" <- w52
          n31 = call "Close.vi"("error in (no error)"=w66, "VISA resource name"=w64) -> ("error out"=w59:errorcluster)  [unwired: 9 in]
          n32 = call "GetSlopeConductance3.vi"("CapacitanceRecords"=w52, "Array in"=w55) -> ("CleanedIV"=→"XY Graph 2":cluster{dbl[], dbl[]}[], "InfoCluster"=→"InfoCluster":T1)  [unwired: 8 in]
          n33 = Unbundle By Name(w59) -> ("status"=w60:bool)
          n34 = case shown="False" w60 {
            tunnel: w59 -> [_ w71]
            tunnel: w58 -> [w68 w69]
            frame False {
              n35 = call "StatusGood.vi"("Text.Text"="Scan Finished", "String in"=w68) -> ()  [unwired: 10 in]
            }
            frame True {
              n36 = Unbundle By Name(w71) -> ("source"=w70:string)
              n37 = call "StatusError.vi"("Text.Text"=w70, "String in"=w69) -> ()  [unwired: 10 in]
            }
          }
        }
        frame True {
          n38 = Unbundle By Name(w72) -> ("source"=w74:string)
          n39 = call "StatusError.vi"("Text.Text"=w74, "String in"=w73) -> ()  [unwired: 10 in]
        }
      }
      "Waveform Graph" <- "Waveform"
    }
    frame True {
      n40 = Unbundle By Name(w97) -> ("source"=w96:string)
      n41 = call "StatusError.vi"("Text.Text"=w96, "String in"=w98) -> ()  [unwired: 10 in]
    }
  }
